vi "APC_9049_HRL_CreateFilter.vi"(4 "sampling freq: fs 2":dbl=1.0 format="%0.2f", 5 "sampling freq: fs":dbl=1.0 format="%0.2f", 6 "order 2":i32=2, 7 "order":i32=2, 8 "low cutoff freq: fl 2":dbl=0.025 format="%0.3f", 9 "high cutoff freq: fh 2":dbl=0.4 format="%0.3f", 10 "low cutoff freq: fl":dbl=0.025 format="%0.3f", 11 "high cutoff freq: fh":dbl=0.1 format="%0.3f") -> (2 "FilterCoefs":T1={"IIR LowPass"={"filter structure"=enum."IIR 2nd Order", "Reverse Coefficients"=[-1.7786317778245848, 0.8008026466657077], "Forward Coefficients"=[0.005542717210280682, 0.011085434420561363, 0.005542717210280682]}, "IIR HighPass"={"filter structure"=enum."IIR 4th Order", "Reverse Coefficients"=[], "Forward Coefficients"=[]}} {"IIR LowPass"."Forward Coefficients" format="%.4f"; "IIR LowPass"."Reverse Coefficients" format="%.4f"})   [LabVIEW 2020]
uses:
  <vilib>/Analysis/3filter.llb/Filter Passband Type.ctl
  <vilib>/Analysis/3filter.llb/Filter Structure Type.ctl
  <vilib>/Analysis/NI_AALBase.lvlib
panel:
  out "error":i32=-20020
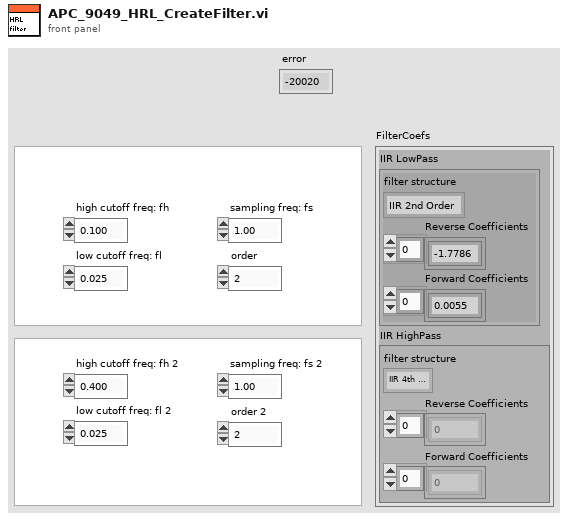
[diagram p1: front panel]
types:
  T1 = cluster{"IIR LowPass":cluster{"filter structure":enum32{"IIR 2nd Order", "IIR 4th Order"}, "Reverse Coefficients":dbl[], "Forward Coefficients":dbl[]}, "IIR HighPass":cluster{"filter structure":enum32{"IIR 2nd Order", "IIR 4th Order"}, "Reverse Coefficients":dbl[], "Forward Coefficients":dbl[]}}
  T2 = typedef "NI_AALBase.lvlib/Filter Structure Type.ctl" = u16
  T3 = typedef "NI_AALBase.lvlib/Filter Passband Type.ctl" = enum32{"Lowpass", "Highpass", "Bandpass", "Bandstop"}
  T4 = cluster{"filter structure":enum32{"IIR 2nd Order", "IIR 4th Order"}, "Reverse Coefficients":dbl[], "Forward Coefficients":dbl[]}
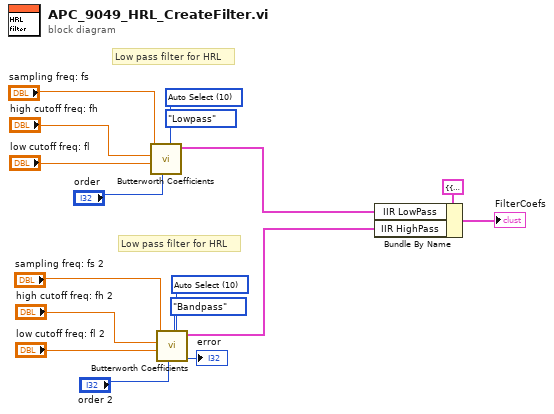
[diagram p0: block diagram]
diagram:
  w6 = T2 10 items=["IIR 2nd Order"=0, "IIR 4th Order"=1, "Auto Select"=10] ("filter structure option")
  w12 = T2 10 items=["IIR 2nd Order"=0, "IIR 4th Order"=1, "Auto Select"=10] ("filter structure option")
  # "Low pass filter for HRL"
  # "Low pass filter for HRL"
  n1 = call <vilib>:"Butterworth Coefficients.vi"("filter structure option"=w12, "order"="order", "filter type"=Filter_Passband_Type."Lowpass", "low cutoff freq: fl"="low cutoff freq: fl", "high cutoff freq: fh"="high cutoff freq: fh", "sampling freq: fs"="sampling freq: fs") -> ("IIR Filter Cluster"=w5:T4)  [unwired: 4 in, 1 out]
  n2 = call <vilib>:"Butterworth Coefficients.vi"("filter structure option"=w6, "order"="order 2", "filter type"=Filter_Passband_Type."Bandpass", "low cutoff freq: fl"="low cutoff freq: fl 2", "high cutoff freq: fh"="high cutoff freq: fh 2", "sampling freq: fs"="sampling freq: fs 2") -> ("error"=→"error":i32, "IIR Filter Cluster"=w4:T4)  [unwired: 4 in]
  n3 = Bundle By Name(cluster=T1 {"IIR LowPass"={"filter structure"=enum."IIR 2nd Order", "Reverse Coefficients"=[-1.7786317778245848, 0.8008026466657077], "Forward Coefficients"=[0.005542717210280682, 0.011085434420561363, 0.005542717210280682]}, "IIR HighPass"={"filter structure"=enum."IIR 2nd Order", "Reverse Coefficients"=[], "Forward Coefficients"=[]}} ("FilterCoefs"), "IIR LowPass"=w5, "IIR HighPass"=w4) -> (→"FilterCoefs":T1)
